vi "globals.vi"() -> ()   [LabVIEW 2017]
panel:
  in  "setPos":bool
  in  "Disconnected":bool
  in  "Authenticated":bool
  in  "Armed":bool
  in  "Dead":bool
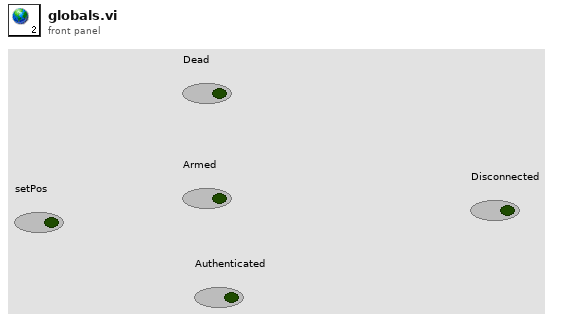
[diagram p1: front panel]
diagram:
